vi "Flatten to CSV Record.vi"(6 "regular expression - protected characters ([])":string="[]", 7 "delimiter (,)":string=",", 10 "error in (no error)":errorcluster, 11 "row of strings":string[](array[string])) -> (2 "error out":errorcluster, 3 "CSV record":string, 5 "can be indented?":bool)   [LabVIEW 2019, in "infolib.lvlib"]
doc: "Convert 1D array of ANSI strings into a single CSV record (row).\n\nThe output CSV record string is formatted in accordance with RFC-4180 (see <b>http://tools.ietf.org/html/rfc4180</b>). \n\nAll cells containing <b>double quotes</b> (0x22), <b>CR</b> (0x0D) , <b>LF</b> (0x0A) or the <b>delimiter character</b> will be enclosed in double quotes. All <b>double quote</b> characters within a cell will be escaped using a second double quote character.\n\nUser can set other <b>protected characters</b> using input \"protected characters regular expression ([])\". Cells containing protected characters will be enclosed in double quotes. Input is regular expression as used in vi \"Match Pattern\". Therefore input \"[]\" matches no characters, input \"\" match all characters, input \"Z\" match character Z, input \"[aBZ]\" match a or B or Z. See help of \"Match Pattern\" for more details.\n\nRev. 0.0 2014-02-20 Ryan Porter\n- First Draft\n\nRev 0.1 2014-10-30 Ryan Porter\n- Convert all CRLF and CR within a cell to LF\n- Changed end of record to CRLF for compatibility with Excel CSV import/export\n\nRev 0.2 2017-01-03 modified for infolib\n\nRev 0.3 2019-04-17 added protected characters"
uses:
  infolib.lvlib
  <vilib>/Utility/error.llb/whitespace.ctl
panel:
  # "Flatten to CSV Record.vi\n\nConvert 1D array of ANSI strings into a single CSV record (row). The output CSV record string is formatted in accordance with RFC-4180 (see http://tools.ietf.org/html/rfc4180). \n\nAll cells containing double quotes (0x22), CR (0x0D) , LF (0x0A) or the delimiter character will be enclosed in double quotes. All double quote characters within a cell will be escaped using a second double quote character. A CRLF is appended to the end of the record."
  # "License: BSD (2-Clause) - http://opensource.org/licenses/BSD-2-Clause \n\nCopyright (c) 2014, Ryan Porter\nAll rights reserved."
  # "Robust CSV v1.1.0\n\nCopyright © 2014, Ryan Porter\nAll rights reserved.\n\nAuthor:\t Ryan Porter\nLAVA Name: Porter\nContact Info:\tContact via PM on lavag.org\n\nLabVIEW Versions:\nLV 2013 (Windows)\nLV 2012 (Windows)\nLV 8.6 (Windows)\n\nDependencies:\nLAVA Palette\n\nDescription:\nThis package contains VIs for reading and writing to CSV files that follow the CSV format outlined in RFC-4180 (see http://tools.ietf.org/html/rfc4180). Using this package, you can properly import CSV files that were exported from spreadsheet programs such as Microsoft Excel, Open Office or LibreOffice Calc as well as export CSV files that will be compatible with any program capable of interpreting CSV files.\n \nThis implementation of the CSV format is capable of handling escaped fields such as those containing commas (or other field delimiters), multiple lines, and double quotes.\n\nInstallation and instructions:\nInstall VIP package using JKI VI Package Manager.\n\nExamples:\n\"<LabVIEW>\\examples\\LAVA\\Robust CSV\\Robust CSV Example Usage.vi\"\tDemonstrates usage of the Read CSV and Write CSV file.\n\nKnown Issues:\nnone\n\nAcknowledgements:\nPhillip Brooks: \"Parse CSV String.vi\" is a modified version of his \"CSV Data File Parser.vi\". His method of parsing the CSV string was much more efficient than my original implementation.\n\nVersion History:\nv1.0.0: Initial release of the code.\nv1.0.1: Modified \"Flatten to CSV Record.vi\" to play nice with Excel CSV import when multi-line cells are present.\nv1.1.0: Moved to LAVA palette & built to VI package file.\n\nLicense:\nDistributed under the BSD 2-Clause (http://opensource.org/licenses/BSD-2-Clause)\nSee link for a full description of the license.\n\nSupport:\nIf you have any problems with this code or want to suggest features go to lavag.org and Navigate to LAVA > Resources > Code Repository (Certified) and\nsearch for the \"Robust CSV\" support page. Or try this link: http://lavag.org/files/file/239-robust-csv/\n\nDistribution:\nThis code was downloaded from the LAVA Code Repository found at lavag.org"
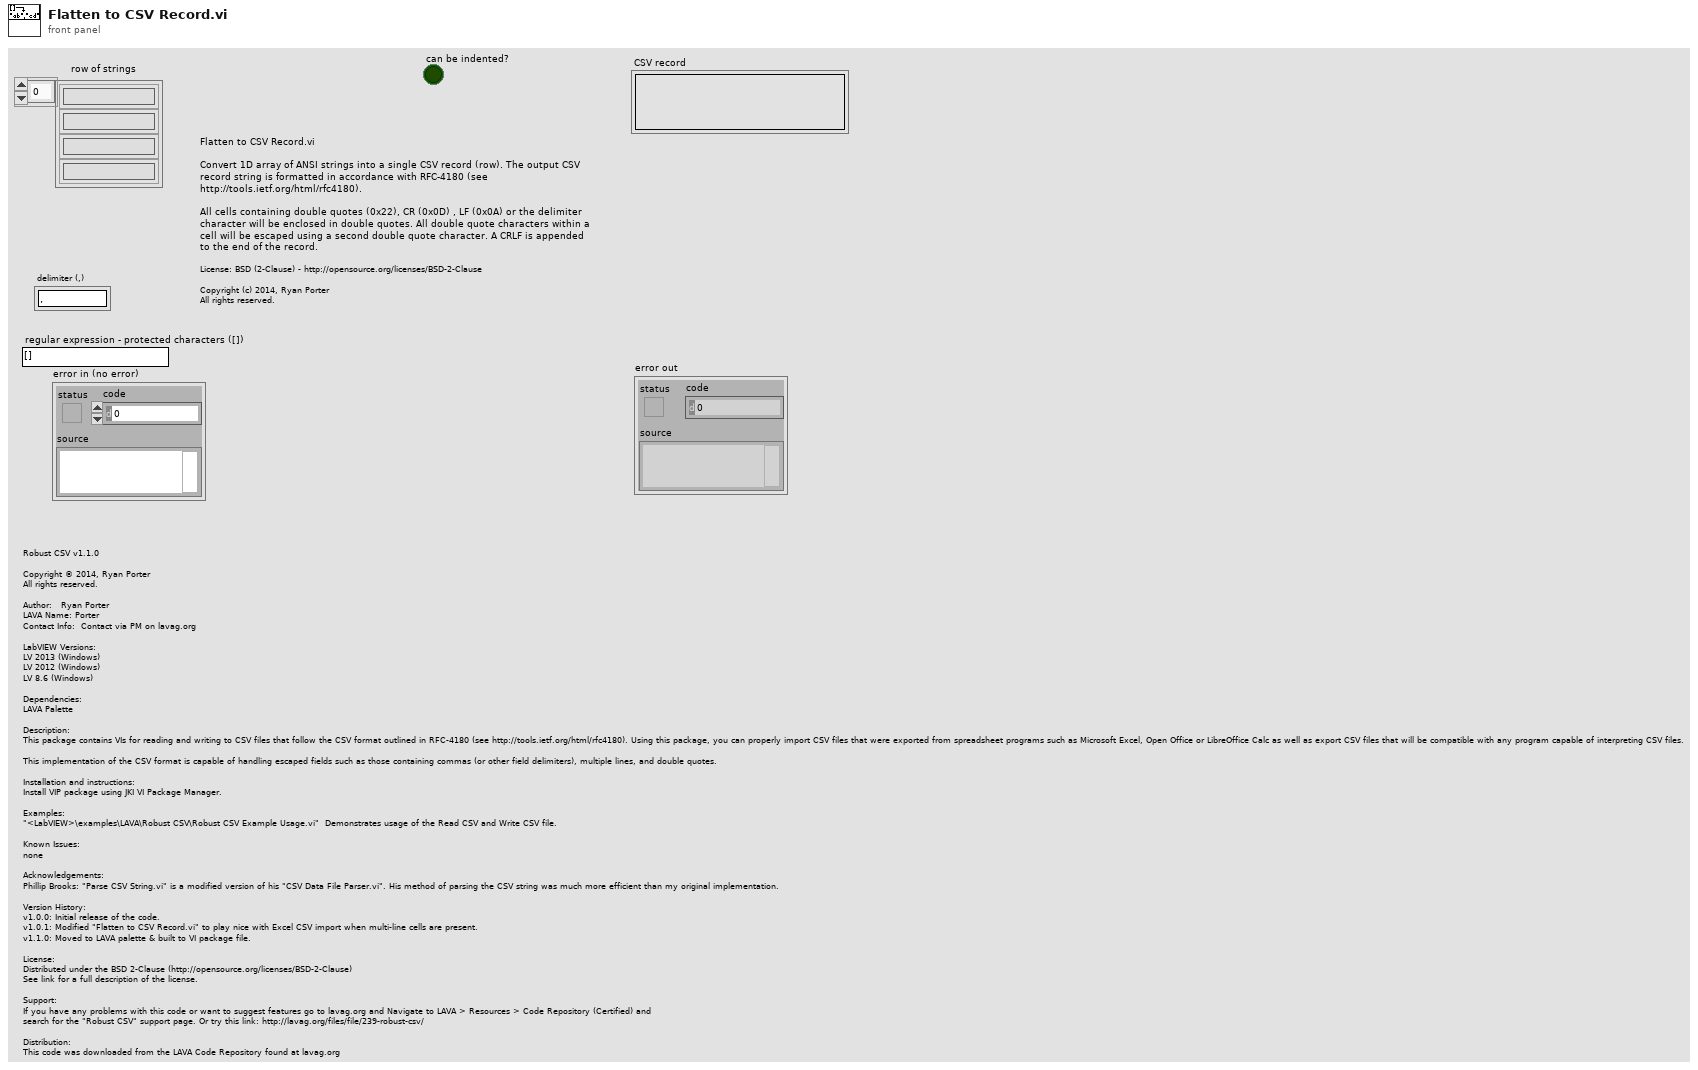
[diagram p1: front panel]
types:
  T1 = typedef "whitespace.ctl" = u16
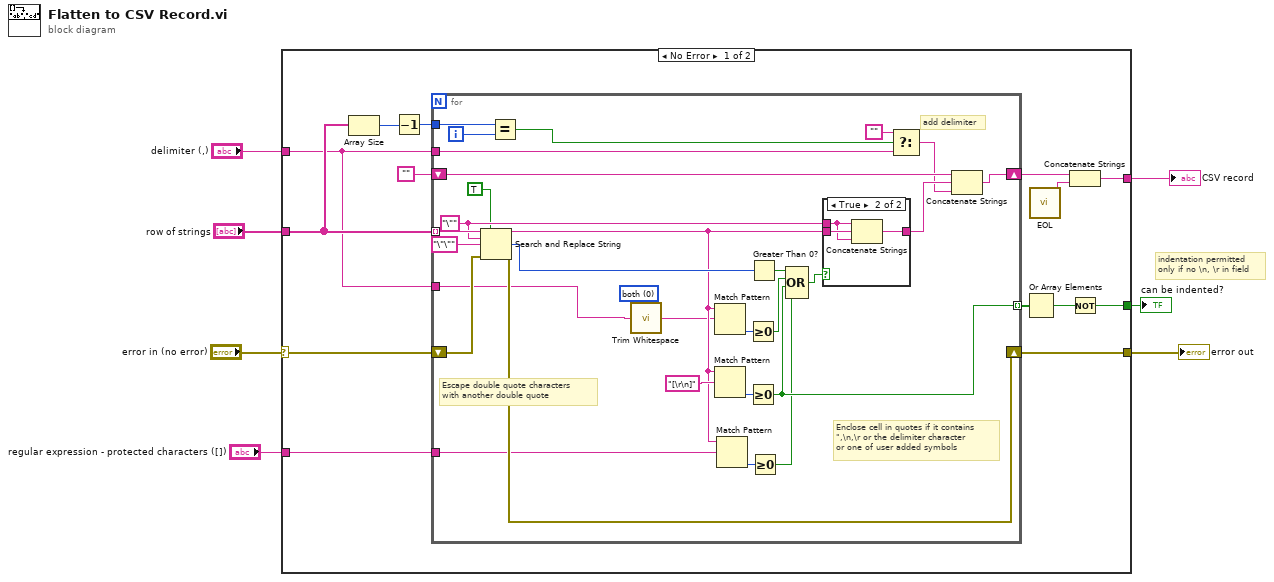
[diagram p0: block diagram]
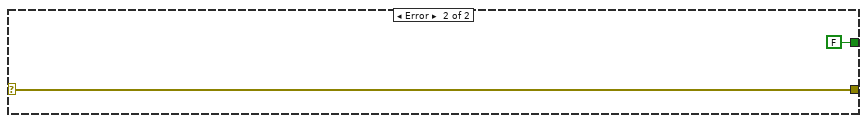
[diagram p3: hidden frame]
diagram:
  # "indentation permitted\nonly if no \\n, \\r in field"
  n1 = case shown="No Error" "error in (no error)" {
    selector: "error in (no error)" -> [w15 w57]
    tunnel: "row of strings" -> [w19 _]
    tunnel: "delimiter (,)" -> [w12 _]
    tunnel: [w16 _] -> w5
    tunnel: [w14 w57] -> w3
    tunnel: [w9 FALSE] -> w2
    tunnel: "regular expression - protected characters ([])" -> [w8 _]
    frame No Error {
      n2 = Array Size(array=w19) -> (size(s)=w18:i32)
      n3 = Decrement(x=w18) -> (x-1=w20:i32)
      n4 = for {
        tunnel: w19 -> [w51] mode=indexing
        shift-right: [w48] -> w17
        shift-left: "" -> [w47]
        tunnel: w12 -> [w42]
        tunnel: w20 -> [w39]
        shift-right: [w31] -> w14
        shift-left: w15 -> [w36]
        tunnel: [w29] -> w13 mode=indexing
        tunnel: w12 -> [w24]
        tunnel: w8 -> [w26]
        i -> [w44]
        w22 = T1 0 items=["both", "start of string", "end of string"] ("location (both)")
        w49 = "\"" ("search string")
        # "Escape double quote characters\nwith another double quote"
        # "Enclose cell in quotes if it contains\n\",\\n,\\r or the delimiter character\nor one of user added symbols"
        # "add delimiter"
        n5 = Search and Replace String(replace all?=TRUE ("replace all? (F)"), input string=w51, search string=w49, replace string="\"\"" ("replace string (\"\")"), error in=w36) -> (result string=w25:string, number of replacements=w38:i32, error out=w31:errorcluster)  [unwired: 4 out]
        n6 = Equal?(x=w39, y=w44) -> (x = y?=w43:bool)
        n7 = call <vilib>:"Trim Whitespace.vi"("string"=w24, "location (both)"=w22) -> ("trimmed string"=w23:string)
        n8 = Match Pattern(string=w25, regular expression=w23) -> (offset past match=w45:i32)  [unwired: 4 out]
        n9 = Match Pattern(string=w25, regular expression="[\r\n]") -> (offset past match=w33:i32)  [unwired: 4 out]
        n10 = Match Pattern(string=w25, regular expression=w26) -> (offset past match=w28:i32)  [unwired: 4 out]
        n11 = Greater Or Equal To 0?(x=w45) -> (x >= 0?=w30:bool)
        n12 = Greater Or Equal To 0?(x=w33) -> (x >= 0?=w29:bool)
        n13 = Greater Than 0?(x=w38) -> (x > 0?=w34:bool)
        n14 = Greater Or Equal To 0?(x=w28) -> (x >= 0?=w27:bool)
        n15 = Compound Arithmetic op=OR(w34, w30, w29, w27) -> (w37:bool)
        n16 = case shown="True" w37 {
          tunnel: w25 -> [w52 w55]
          tunnel: w49 -> [_ w54]
          tunnel: [w52 w53] -> w46
          frame False {
          }
          frame True {
            n17 = Concatenate Strings(w54, w55, w54) -> (w53:string)
          }
        }
        n18 = Select(t="", s=w43, f=w42) -> (s? t:f=w40:string)
        n19 = Concatenate Strings(w47, w46, w40) -> (w48:string)
      }
      n20 = Or Array Elements(Boolean array=w13) -> (logical OR=w10:bool)
      n21 = call "EOL.vi"() -> ("eol"=w11:string)  [unwired: 11 in]
      n22 = Concatenate Strings(w17, w11) -> (w16:string)
      n23 = Not(x=w10) -> (.not. x?=w9:bool)
    }
    frame Error {
    }
  }
  "CSV record" <- w5
  "error out" <- w3
  "can be indented?" <- w2
